vi "TestLoader_Init.vi"(8 "error in (no error)":errorcluster, 11 "TestLoader in":refnum<class "TestLoader.lvclass">) -> (0 "error out":errorcluster, 3 "TestLoader out":refnum<class "TestLoader.lvclass">)   [LabVIEW 2013, in "TestLoader.lvclass"]
uses:
  TestLoader.lvclass
  TestLoader.lvclass/TestLoader.ctl
panel:
  # "JKI VI Tester for LabVIEW\nhttp://jkisoft.com/vi-tester\nCopyright (C) 2007-2009, JKI <info@jkisoft.com>\nALL RIGHTS RESERVED"
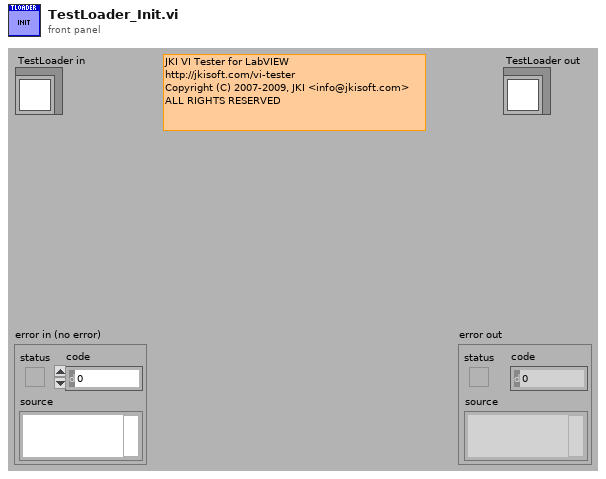
[diagram p1: front panel]
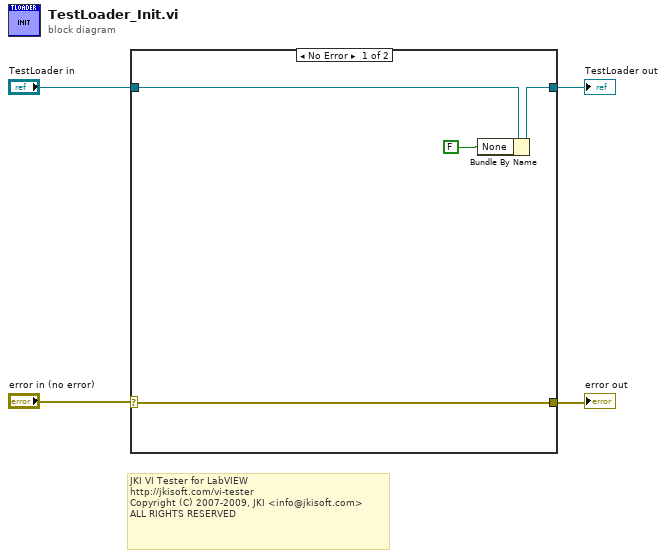
[diagram p0: block diagram]
diagram:
  # "JKI VI Tester for LabVIEW\nhttp://jkisoft.com/vi-tester\nCopyright (C) 2007-2009, JKI <info@jkisoft.com>\nALL RIGHTS RESERVED"
  n1 = case shown="No Error" "error in (no error)" {
    selector: "error in (no error)" -> [w5 w9]
    tunnel: "TestLoader in" -> [w8 w10]
    tunnel: [w7 w10] -> w3
    tunnel: [w5 w9] -> w1
    frame No Error {
      n2 = Bundle By Name(cluster=w8, "None"=FALSE) -> (w7:refnum<class "TestLoader.lvclass">)
    }
    frame Error {
    }
  }
  "TestLoader out" <- w3
  "error out" <- w1
